vi "Derivadas_Integral.vi"() -> ()   [LabVIEW 2017]
panel:
  out "XY Graph 3":cluster{dbl[], dbl[]}(graph)
  out "XY Graph 2":cluster{dbl[], dbl[]}(graph)
  out "XY Graph":cluster{dbl[], dbl[]}(graph)
  in  "df":dbl
  in  "to":dbl
  in  "tf":dbl
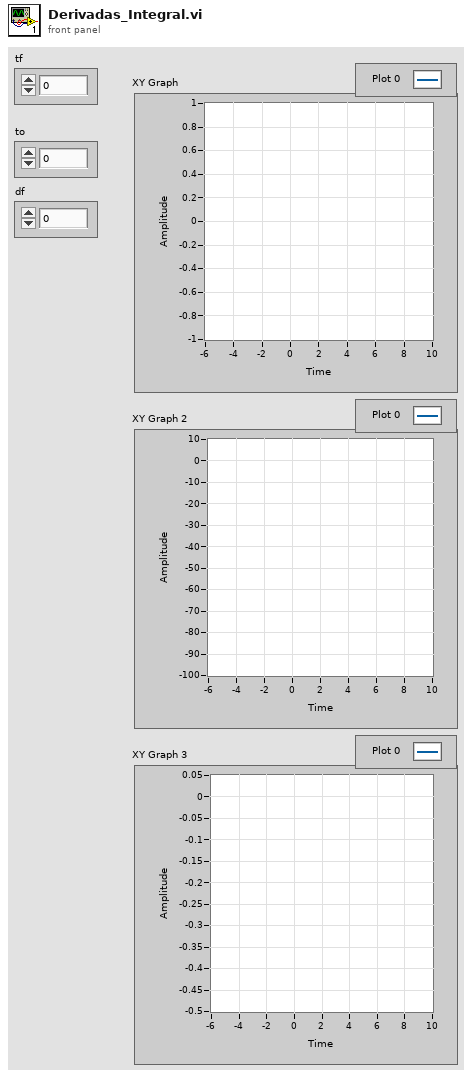
[diagram p1: front panel]
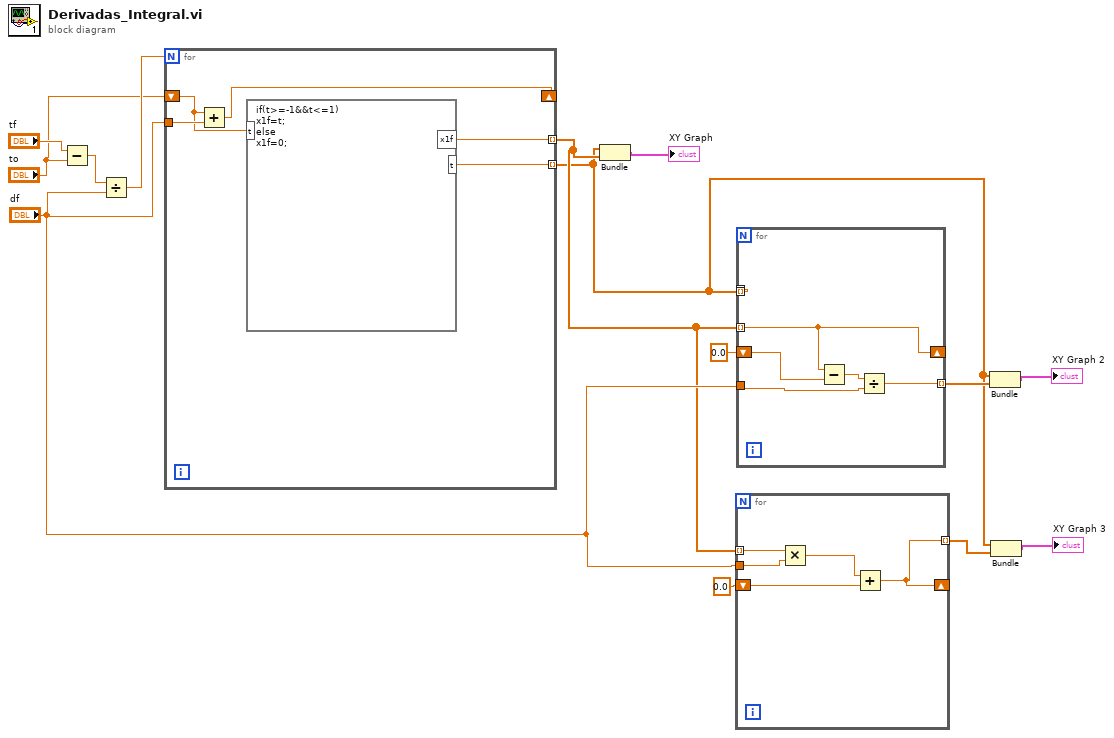
[diagram p0: block diagram]
diagram:
  n1 = Subtract(x="tf", y="to") -> (x-y=w13:dbl)
  n2 = Divide(x=w13, y="df") -> (x/y=w12:dbl)
  n3 = for {
    N: w12 -> [_]
    shift-right: [w19] -> _
    shift-left: "to" -> [w17]
    tunnel: "df" -> [w18]
    tunnel: [w16] -> w5 mode=indexing
    tunnel: [w15] -> w2 mode=indexing
    n4 = Add(x=w17, y=w18) -> (x+y=w19:dbl)
    n5 = formula code="if(t>=-1&&t<=1)\nx1f=t;\nelse\nx1f=0;"("t"=w17) -> ("x1f"=w16:dbl, "t"=w15:dbl)
  }
  n6 = Bundle(w2, w5) -> (→"XY Graph":cluster{dbl[], dbl[]})  [unwired: 1 in]
  n7 = for {
    tunnel: "df" -> [w24]
    tunnel: w5 -> [w23] mode=indexing
    shift-right: [w20] -> _
    shift-left: 0.0 -> [w21]
    tunnel: [w20] -> w1 mode=indexing
    n8 = Multiply(x=w23, y=w24) -> (x*y=w22:dbl)
    n9 = Add(x=w22, y=w21) -> (x+y=w20:dbl)
  }
  n10 = for {
    tunnel: [w30] -> _ mode=indexing
    tunnel: w2 -> [w30] mode=indexing
    shift-right: [w25] -> _
    shift-left: 0.0 ("x1f") -> [w29]
    tunnel: "df" -> [w27]
    tunnel: [w26] -> w8 mode=indexing
    tunnel: w5 -> [w25] mode=indexing
    n11 = Subtract(x=w25, y=w29) -> (x-y=w28:dbl)
    n12 = Divide(x=w28, y=w27) -> (x/y=w26:dbl)
  }
  n13 = Bundle(w2, w8) -> (→"XY Graph 2":cluster{dbl[], dbl[]})  [unwired: 1 in]
  n14 = Bundle(w2, w1) -> (→"XY Graph 3":cluster{dbl[], dbl[]})  [unwired: 1 in]
